vi "DSF.Engine.Framework.Create.Plugins.vi"(8 "error in (no error)":errorcluster, 10 "Plugin Configurations":refnum<class "DSF.Shared.Configuration.Plugin.lvclass">[](array[class]), 11 "Framework in":refnum<class "DSF.Engine.Framework.lvclass">) -> (0 "error out":errorcluster, 2 "Plugins":refnum<class "DSF.Engine.Plugin.lvclass">[](array[class]), 3 "Framework out":refnum<class "DSF.Engine.Framework.lvclass">)   [LabVIEW 2017, in "DSF.Engine.lvlib" / "DSF.Engine.Framework.lvclass"]
uses:
  DSF.Engine.Framework.lvclass
  Shared/Classes/Plugin/DSF.Shared.Configuration.Plugin.lvclass
  Plugin/DSF.Engine.Plugin.lvclass
  DSF.Engine.Framework.lvclass/DSF.Engine.Framework.ctl
  Shared/Classes/Plugin/DSF.Shared.Configuration.Plugin.lvclass/DSF.Shared.Configuration.Plugin.ctl
  Transceiver/DSF.Engine.Transceiver.lvclass
  Timing/DSF.Engine.Timing.lvclass
  Transceiver/DSF.Engine.Transceiver Loader.lvclass
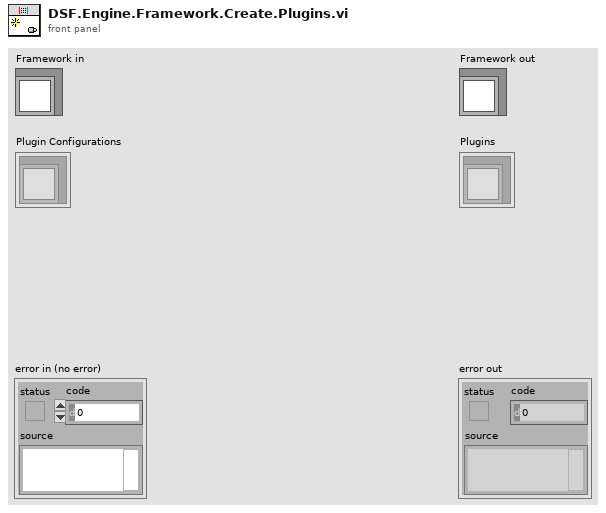
[diagram p1: front panel]
types:
  T1 = typedef "DSF Configuration API.lvlib/DSF Timing Info.ctl" = cluster{"priority":u64, "decimation":u64, "offset":u64}
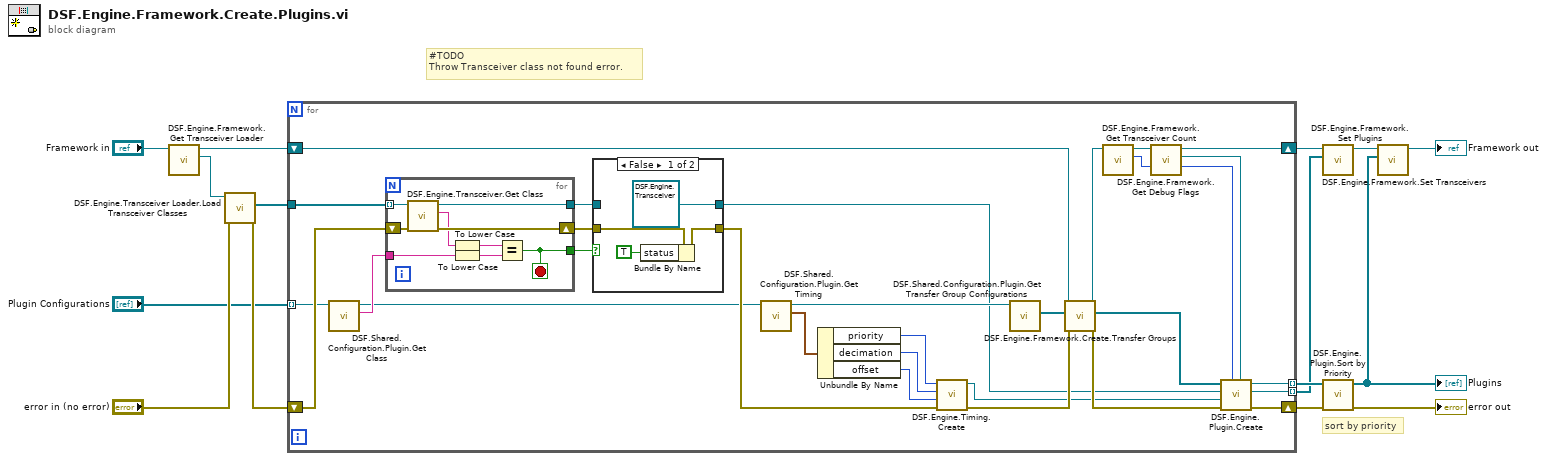
[diagram p0: block diagram]
diagram:
  # "#TODO\nThrow Transceiver class not found error."
  # "sort by priority"
  n1 = call "DSF.Engine.Framework.Get Transceiver Loader.vi"("Framework in"="Framework in") -> ("Transceiver Loader"=w6:refnum<class "DSF.Engine.Transceiver Loader.lvclass">, "Framework out"=w7:refnum<class "DSF.Engine.Framework.lvclass">)  [unwired: 9 in]
  n2 = call "DSF.Engine.Transceiver Loader.Load Transceiver Classes.vi"("error in (no error)"="error in (no error)", "Transceiver Loader in"=w6) -> ("error out"=w3:errorcluster, "Transceivers"=w5:refnum<class "DSF.Engine.Transceiver.lvclass">[])  [unwired: 7 in, 1 out]
  n3 = for {
    shift-right: [w40] -> w14
    shift-left: w3 -> [w22]
    shift-right: [w34] -> w10
    shift-left: w7 -> [w38]
    tunnel: "Plugin Configurations" -> [w20] mode=indexing
    tunnel: [w36] -> w12 mode=indexing
    tunnel: [w28] -> w1 mode=indexing
    tunnel: w5 -> [w26]
    n4 = call "DSF.Shared.Configuration.Plugin.Get Class.vi"("Plugin Configuration in"=w20) -> ("class"=w25:string, "Plugin Configuration out"=w19:refnum<class "DSF.Shared.Configuration.Plugin.lvclass">)  [unwired: 9 in]
    n5 = for {
      tunnel: w26 -> [w59] mode=indexing
      tunnel: w25 -> [w58]
      tunnel: [w55] -> w18
      tunnel: [w54] -> w24
      shift-right: [w52] -> w23
      shift-left: w22 -> [w53]
      stop <- w54 stop-if-true
      n6 = call-dynamic "DSF.Engine.Transceiver.Get Class.vi"("error in (no error)"=w53, "Transceiver in"=w59) -> ("error out"=w52:errorcluster, "class"=w51:string, "Transceiver out"=w55:refnum<class "DSF.Engine.Transceiver.lvclass">)  [unwired: 7 in]
      n7 = To Lower Case(string=w51) -> (all lower case string=w56:string)
      n8 = To Lower Case(string=w58) -> (all lower case string=w57:string)
      n9 = Equal?(x=w56, y=w57) -> (x = y?=w54:bool)
    }
    n10 = case shown="False" w24 {
      tunnel: w23 -> [w48 w50]
      tunnel: [w46 w50] -> w21
      tunnel: w18 -> [_ w49]
      tunnel: [refnum<class "DSF.Engine.Transceiver.lvclass"> refnum ("Transceiver out") w49] -> w16
      frame False {
        n11 = Bundle By Name(cluster=w48, "status"=TRUE) -> (w46:errorcluster)
      }
      frame True {
      }
    }
    n12 = call "DSF.Shared.Configuration.Plugin.Get Timing.vi"("Plugin Configuration in"=w19) -> ("cycle timing"=w44:T1, "Plugin Configuration out"=w27:refnum<class "DSF.Shared.Configuration.Plugin.lvclass">)  [unwired: 9 in]
    n13 = Unbundle By Name(w44) -> ("priority"=w41:u64, "decimation"=w42:u64, "offset"=w43:u64)
    n14 = call "DSF.Engine.Timing.Create.vi"("error in (no error)"=w21, "Offset"=w43, "Decimation"=w42, "Priority"=w41) -> ("error out"=w37:errorcluster, "Timing"=w29:refnum<class "DSF.Engine.Timing.lvclass">)  [unwired: 6 in]
    n15 = call "DSF.Shared.Configuration.Plugin.Get Transfer Group Configurations.vi"("Plugin Configuration in"=w27) -> ("Transfer Group Configurations"=w39:refnum<class "DSF.Shared.Configuration.Transfer Group.lvclass">[])  [unwired: 9 in, 1 out]
    n16 = call "DSF.Engine.Framework.Create.Transfer Groups.vi"("error in (no error)"=w37, "Transfer Group Configurations"=w39, "Framework in"=w38) -> ("error out"=w30:errorcluster, "Transfer Groups"=w31:refnum<class "DSF.Engine.Transfer Group.lvclass">[], "Framework out"=w35:refnum<class "DSF.Engine.Framework.lvclass">)  [unwired: 6 in]
    n17 = call "DSF.Engine.Framework.Get Transceiver Count.vi"("Framework in"=w35) -> ("transceiver count"=w17:i32, "Framework out"=w33:refnum<class "DSF.Engine.Framework.lvclass">)  [unwired: 9 in]
    n18 = call "DSF.Engine.Framework.Get Debug Flags.vi"("Framework in"=w33) -> ("Debug Flags"=w32:refnum<class "DSF.Engine.Debug Flags.lvclass">, "Framework out"=w34:refnum<class "DSF.Engine.Framework.lvclass">)  [unwired: 9 in]
    n19 = call "DSF.Engine.Plugin.Create.vi"("Debug Flags"=w32, "transceiver count"=w17, "error in (no error)"=w30, "Timing"=w29, "Transceiver type"=w16, "Transfer Groups"=w31) -> ("error out"=w40:errorcluster, "Transceiver"=w28:refnum<class "DSF.Engine.Transceiver.lvclass">, "Plugin out"=w36:refnum<class "DSF.Engine.Plugin.lvclass">)  [unwired: 3 in]
  }
  n20 = call "DSF.Engine.Framework.Set Transceivers.vi"("Transceivers"=w1, "Framework in"=w10) -> ("Framework out"=w9:refnum<class "DSF.Engine.Framework.lvclass">)  [unwired: 9 in]
  n21 = call "DSF.Engine.Plugin.Sort by Priority.vi"("error in (no error)"=w14, "Plugins in"=w12) -> ("error out"=→"error out":errorcluster, "Plugins out"=w11:refnum<class "DSF.Engine.Plugin.lvclass">[])  [unwired: 8 in]
  "Plugins" <- w11
  n22 = call "DSF.Engine.Framework.Set Plugins.vi"("Plugins"=w11, "Framework in"=w9) -> ("Framework out"=→"Framework out":refnum<class "DSF.Engine.Framework.lvclass">)  [unwired: 9 in]
